vi "ParseOptions.vi"(8 "error in (no error)":errorcluster, 10 "Options":string[](array[string]), 11 "Restore in":refnum<class "Restore.lvclass">) -> (0 "error out":errorcluster, 3 "Restore out":refnum<class "Restore.lvclass">)   [LabVIEW 2014, in "Restore.lvclass"]
uses:
  Restore.lvclass
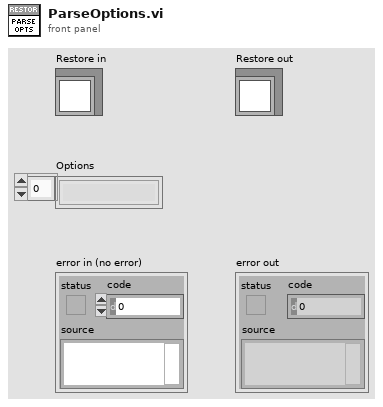
[diagram p1: front panel]
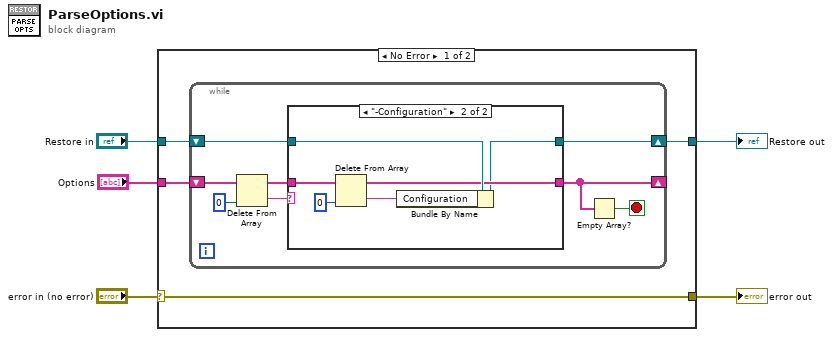
[diagram p0: block diagram]
diagram:
  n1 = case shown="No Error" "error in (no error)" {
    selector: "error in (no error)" -> [w9 w27]
    tunnel: [w9 w27] -> w3
    tunnel: [w7 w26] -> w4
    tunnel: "Restore in" -> [w6 w26]
    tunnel: "Options" -> [w8 _]
    frame No Error {
      n2 = while {
        shift-right: [w13] -> _
        shift-left: w8 -> [w17]
        shift-right: [w11] -> w7
        shift-left: w6 -> [w10]
        stop <- w12 stop-if-true
        n3 = Delete From Array(array=w17, index=0) -> (deleted portion=w15:string, array with subset deleted=w14:string[])  [unwired: 1 in]
        n4 = case shown="\"-Configuration\"" w15 {
          tunnel: [w19 w23] -> w13
          tunnel: w14 -> [w19 w24]
          tunnel: [w18 w21] -> w11
          tunnel: w10 -> [w18 w25]
          frame Default {
          }
          frame "-Configuration" {
            n5 = Delete From Array(array=w24, index=0) -> (deleted portion=w20:string, array with subset deleted=w23:string[])  [unwired: 1 in]
            n6 = Bundle By Name(cluster=w25, "Configuration"=w20) -> (w21:refnum<class "Restore.lvclass">)
          }
        }
        n7 = Empty Array?(array=w13) -> (empty?=w12:bool)
      }
    }
    frame Error {
    }
  }
  "error out" <- w3
  "Restore out" <- w4
